vi "Elipse Finder Using Resize.vi"(6 "Zoom Image":T1, 7 "X":u16, 8 "EndRadius":u16, 9 "StartRadius":u16, 10 "Y":u16, 11 "Refnum in":T1) -> (0 "MaxA":dbl, 1 "MaxB":dbl, 2 "MaxX":dbl, 3 "MaxY":dbl, 4 "transposed array":u8[][](graph), 5 "MaxGrade":u32)   [LabVIEW 2015]
uses:
  <vilib>/vision/Image Controls.llb/IMAQ Image.ctl
  Controls/Pivot Finder Input Params Typedef.ctl
  <vilib>/vision/NI_Vision_Development_Module.lvlib
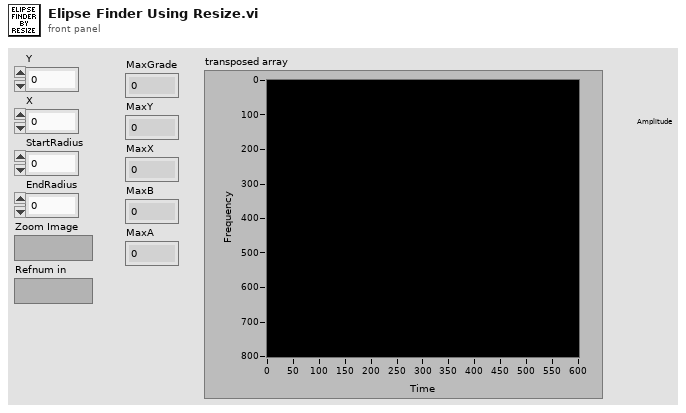
[diagram p1: front panel]
types:
  T1 = typedef "IMAQ Image.ctl" = refnum<image>
  T2 = typedef "Pivot Finder Input Params Typedef.ctl" = cluster{"Ymin":u32, "Ymax":u32, "Xmin":u32, "Xmax":u32, "Amin":u32, "Amax":u32, "Bmin":u32, "Bmax":u32}
  T3 = cluster{"Left":i32, "Top":i32, "Right":i32, "Bottom":i32}
  T4 = cluster{"Ymin":dbl, "Ymax":dbl, "Xmin":dbl, "Xmax":dbl, "Amin":dbl, "Amax":dbl, "Bmin":dbl, "Bmax":dbl}
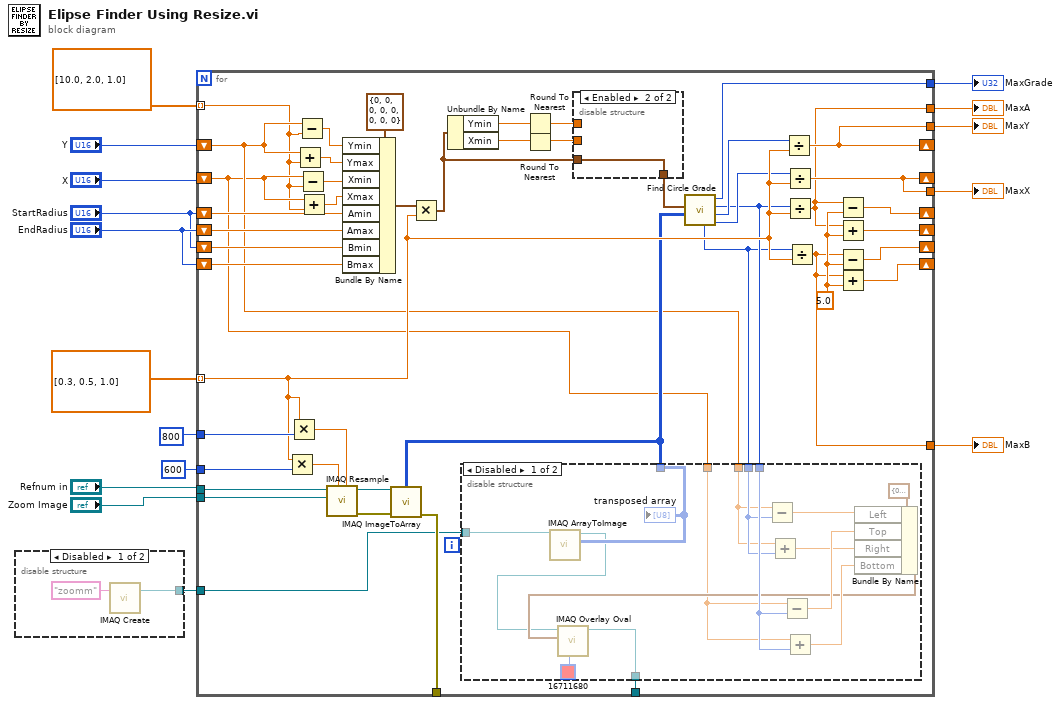
[diagram p0: block diagram]
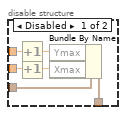
[diagram p3: hidden frame]
diagram:
  n1 = disable-structure shown="Disabled" {
    disable-tunnel: [w18 _] -> w7
    frame Disabled {
      n2 = call "IMAQ Create"("Image Name"="zoomm") -> ("New Image"=w18:T1)  [unwired: 3 in, 2 out]
    }
    frame Enabled {
    }
  }
  n3 = for {
    tunnel: "Zoom Image" -> [w62]
    tunnel: "Refnum in" -> [w63]
    tunnel: dbl[] [0.3, 0.5, 1.0] -> [w54] mode=indexing
    tunnel: 800 -> [w61]
    tunnel: 600 -> [w60]
    shift-right: [w40] -> _
    shift-left: "Y" -> [w23]
    shift-right: [w39] -> _
    shift-left: "X" -> [w21]
    shift-right: [w50] -> _
    shift-left: "StartRadius" -> [w53]
    shift-right: [w49] -> _
    shift-left: "EndRadius" -> [w56]
    shift-right: [w46] -> _
    shift-left: "StartRadius" -> [w52]
    shift-right: [w48] -> _
    shift-left: "EndRadius" -> [w51]
    tunnel: [w45] -> _
    tunnel: [w36] -> w8
    tunnel: [w39] -> w5
    tunnel: [w37] -> w9
    tunnel: [w40] -> w4
    tunnel: w7 -> [w33]
    tunnel: [w29] -> w14
    tunnel: [w28] -> _
    tunnel: dbl[] [10.0, 2.0, 1.0] -> [w19] mode=indexing
    w47 = 5.0 ("y")
    n4 = Multiply(x=w54, y=w60) -> (x*y=w59:dbl)
    n5 = Multiply(x=w54, y=w61) -> (x*y=w58:dbl)
    n6 = Add(x=w23, y=w19) -> (x+y=w25:dbl)
    n7 = Subtract(x=w23, y=w19) -> (x-y=w24:dbl)
    n8 = Subtract(x=w21, y=w19) -> (x-y=w27:dbl)
    n9 = Add(x=w21, y=w19) -> (x+y=w26:dbl)
    n10 = call "IMAQ Resample"("X Resolution"=w58, "Y Resolution"=w59, "Image Dst"=w62, "Image Src"=w63) -> ("error out"=w64:errorcluster, "Image Dst Out"=w35:T1)  [unwired: 6 in]
    n11 = Bundle By Name(cluster=T2 {"Ymin"=0, "Ymax"=0, "Xmin"=0, "Xmax"=0, "Amin"=0, "Amax"=0, "Bmin"=0, "Bmax"=0} ("Cluster"), "Ymin"=w24, "Ymax"=w25, "Xmin"=w27, "Xmax"=w26, "Amin"=w53, "Amax"=w56, "Bmin"=w52, "Bmax"=w51) -> (w55:T2)
    n12 = call "IMAQ ImageToArray"("error in (no error)"=w64, "Image"=w35) -> ("error out"=w45:errorcluster, "Image Pixels (U8)"=w32:u8[][])  [unwired: 2 in, 3 out]
    n13 = Multiply(x=w55, y=w54) -> (x*y=w43:T4)
    n14 = Unbundle By Name(w43) -> ("Ymin"=w34:dbl, "Xmin"=w38:dbl)
    n15 = Round To Nearest(number=w34) -> (nearest integer value=w22:dbl)
    n16 = Round To Nearest(number=w38) -> (nearest integer value=w20:dbl)
    n17 = disable-structure shown="Enabled" {
      disable-tunnel: [w70 w71] -> w44
      disable-tunnel: w43 -> [w67 w71]
      disable-tunnel: w22 -> [w66 _]
      disable-tunnel: w20 -> [w65 _]
      frame Disabled {
        n18 = Increment(x=w66) -> (x+1=w69:dbl)
        n19 = Increment(x=w65) -> (x+1=w68:dbl)
        n20 = Bundle By Name(cluster=w67, "Ymax"=w69, "Xmax"=w68) -> (w70:T4)
      }
      frame Enabled {
      }
    }
    n21 = call "Find Circle Grade.vi"("Picture"=w32, "Cluster"=w44) -> ("MaxX"=w42:u32, "MaxY"=w41:u32, "MaxA"=w31:u32, "MaxGrade"=w29:u32, "MaxB"=w30:u32)  [unwired: 5 in]
    n22 = disable-structure shown="Disabled" {
      disable-tunnel: w33 -> [w86 _]
      disable-tunnel: w32 -> [w85 _]
      disable-tunnel: w31 -> [w84 _]
      disable-tunnel: w30 -> [w83 _]
      disable-tunnel: [w74 _] -> w28
      disable-tunnel: w23 -> [w73 _]
      disable-tunnel: w21 -> [w72 _]
      frame Disabled {
        n23 = call "IMAQ ArrayToImage"("Image Pixels (U8)"=w85, "Image"=w86) -> ("Image Out"=w75:T1)  [unwired: 8 in, 1 out]
        n24 = Subtract(x=w73, y=w83) -> (x-y=w79:dbl)
        n25 = Add(x=w73, y=w83) -> (x+y=w80:dbl)
        n26 = Subtract(x=w72, y=w84) -> (x-y=w81:dbl)
        n27 = Add(x=w72, y=w84) -> (x+y=w82:dbl)
        n28 = Bundle By Name(cluster=T3 {"Left"=0, "Top"=0, "Right"=0, "Bottom"=0} ("Bounding Rectangle"), "Left"=w79, "Top"=w81, "Right"=w80, "Bottom"=w82) -> (w76:T3)
        n29 = call "IMAQ Overlay Oval"("Color"=u32 16711680, "Bounding Rectangle"=w76, "Image"=w75) -> ("Image Out"=w74:T1)  [unwired: 7 in, 1 out]
        "transposed array" <- w85
      }
      frame Enabled {
      }
    }
    n30 = Divide(x=w41, y=w54) -> (x/y=w40:dbl)
    n31 = Divide(x=w42, y=w54) -> (x/y=w39:dbl)
    n32 = Divide(x=w31, y=w54) -> (x/y=w37:dbl)
    n33 = Divide(x=w30, y=w54) -> (x/y=w36:dbl)
    n34 = Subtract(x=w37, y=w47) -> (x-y=w50:dbl)
    n35 = Add(x=w37, y=w47) -> (x+y=w49:dbl)
    n36 = Subtract(x=w36, y=w47) -> (x-y=w46:dbl)
    n37 = Add(x=w36, y=w47) -> (x+y=w48:dbl)
  }
  "MaxGrade" <- w14
  "MaxA" <- w9
  "MaxB" <- w8
  "MaxX" <- w5
  "MaxY" <- w4
